vi "Broadcast Inbound Message.vi"(8 "error in (no error)":errorcluster, 10 "Inbound Message":refnum<class "PUBLISH.lvclass">, 11 "MQTT_Base in":refnum<class "MQTT_Base.lvclass">) -> (0 "error out":errorcluster, 3 "MQTT_Base out":refnum<class "MQTT_Base.lvclass">)   [LabVIEW 2013, in "MQTT Base.lvlib" / "MQTT_Base.lvclass"]
uses:
  MQTT_Base.lvclass
  <vilib>/LabVIEW Open Source Project/MQTT Control Packets/Control Packets/PUBLISH/PUBLISH.lvclass
  MQTT_Base.lvclass/MQTT_Base.ctl
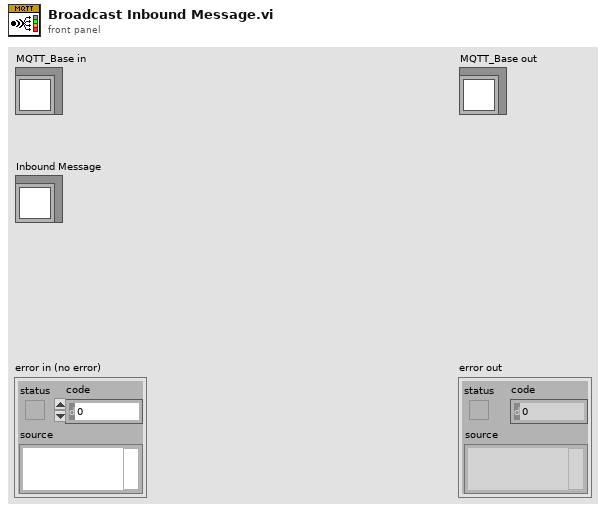
[diagram p1: front panel]
types:
  T1 = typedef "MQTT Base.lvlib/MQTT_Base.lvclass/Public Events -- cluster.ctl" = cluster{"Stop Event":refnum<user-event>, "Error Event":refnum<user-event>, "Inbound Message":refnum<user-event>}
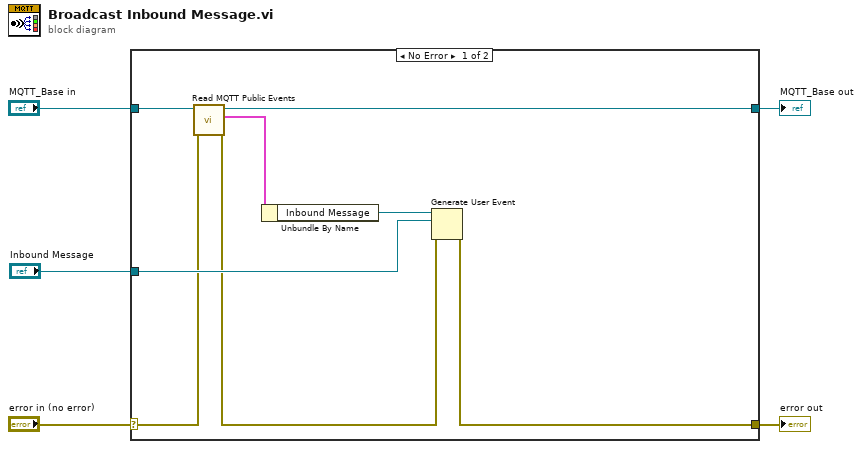
[diagram p0: block diagram]
diagram:
  n1 = case shown="No Error" "error in (no error)" {
    selector: "error in (no error)" -> [w9 w15]
    tunnel: [w13 w15] -> w4
    tunnel: [w6 w14] -> w2
    tunnel: "MQTT_Base in" -> [w7 w14]
    tunnel: "Inbound Message" -> [w12 _]
    frame No Error {
      n2 = call "Read MQTT Public Events.vi"("error in (no error)"=w9, "MQTT_Base in"=w7) -> ("error out"=w8:errorcluster, "MQTT Public Events"=w11:T1, "MQTT_Base out"=w6:refnum<class "MQTT_Base.lvclass">)  [unwired: 7 in]
      n3 = Unbundle By Name(w11) -> ("Inbound Message"=w10:refnum<user-event>)
      n4 = Generate User Event(user event=w10, event data cluster=w12, error in=w8) -> (error out=w13:errorcluster)  [unwired: 1 in, 1 out]
    }
    frame Error {
    }
  }
  "error out" <- w4
  "MQTT_Base out" <- w2
